vi "Lire Datas.vi"(8 "error in (no error)":errorcluster caption="entrée d'erreur (pas d'erreur)", 11 "Share en entrée":refnum<class "Stock.lvclass">) -> (0 "error out":errorcluster caption="sortie d'erreur", 2 "Datas":T1[](array[typedef]), 3 "Share en sortie":refnum<class "Stock.lvclass">)   [LabVIEW 2012, in "Stock.lvclass"]
uses:
  Stock.lvclass
  Stock_Data.ctl
  Stock.lvclass/Stock.ctl
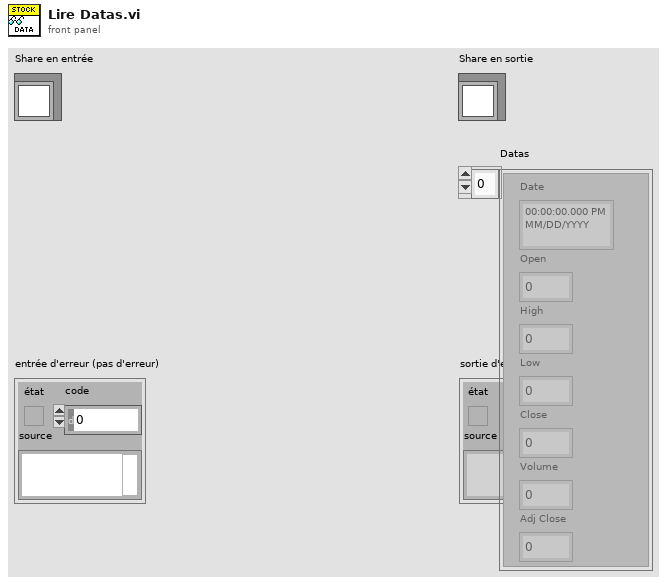
[diagram p1: front panel]
types:
  T1 = typedef "Stock_Data.ctl" = cluster{"Date":timestamp, "Open":dbl, "High":dbl, "Low":dbl, "Close":dbl, "Volume":dbl, "Adj Close":dbl}
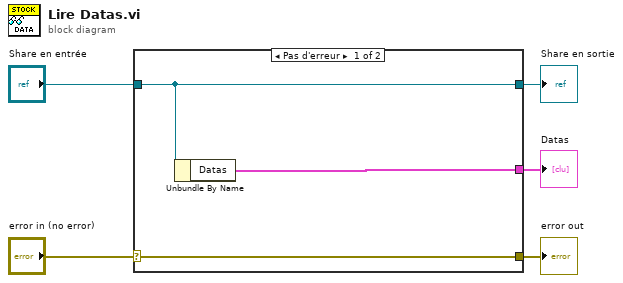
[diagram p0: block diagram]
diagram:
  n1 = case shown="Pas d'erreur" "error in (no error)" {
    selector: "error in (no error)" -> [w8 w9]
    tunnel: [w8 w9] -> w4
    tunnel: [w7 w10] -> w2
    tunnel: "Share en entrée" -> [w7 w10]
    tunnel: [w6 _] -> w1
    frame No Error {
      n2 = Unbundle By Name(w7) -> ("Datas"=w6:T1[])
    }
    frame Error {
    }
  }
  "error out" <- w4
  "Share en sortie" <- w2
  "Datas" <- w1
